vi "test Thermal Chamber Response Simulator_Init-Init.vi"(8 "error in (no error)":errorcluster, 11 "TestCase in":refnum<class "Thermal Chamber Response Simulator_Init.lvclass">) -> (0 "error out":errorcluster, 3 "TestCase out":refnum<class "Thermal Chamber Response Simulator_Init.lvclass">)   [LabVIEW 2018, in "Thermal Chamber Response Simulator_Init.lvclass"]
uses:
  Thermal Chamber Response Simulator_Init.lvclass
  Libraries/Thermal Chamber Response Simulator/Thermal Chamber Response Simulator.lvlib
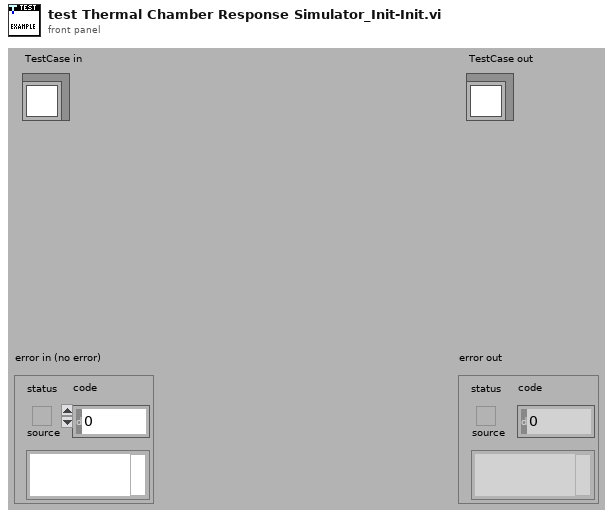
[diagram p1: front panel]
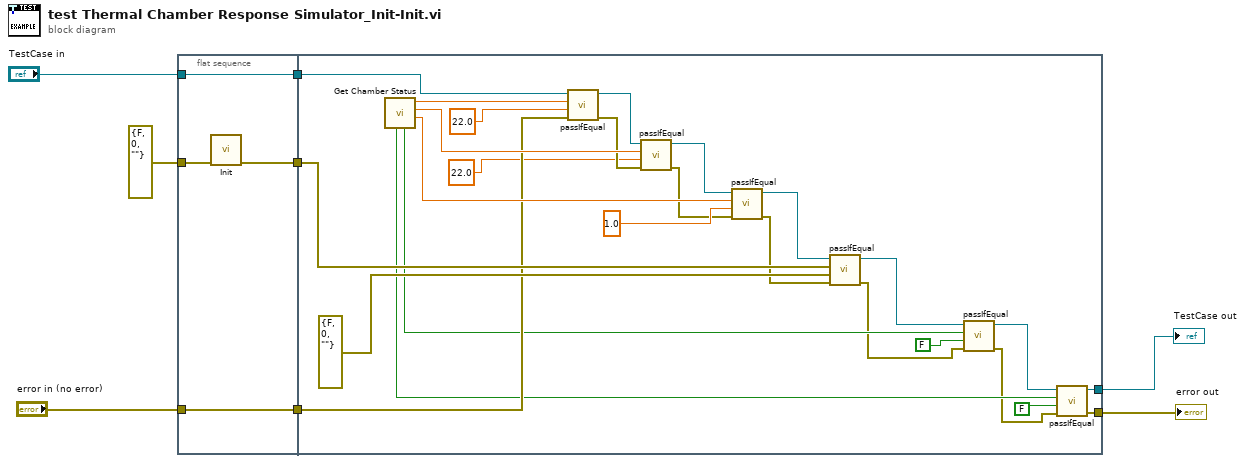
[diagram p0: block diagram]
diagram:
  n1 = flat-sequence {
    tunnel: errorcluster {"status"=FALSE, "code"=0, "source"=""} ("error in (no error)") -> [w12]
    tunnel: [w11] -> w7
    tunnel: "error in (no error)" -> [w10]
    tunnel: [w10] -> w6
    tunnel: [w9] -> w4
    tunnel: "TestCase in" -> [w9]
    tunnel: w7 -> [w38]
    tunnel: w6 -> [w27]
    tunnel: w4 -> [w31]
    tunnel: [w15] -> w2
    tunnel: [w14] -> w1
    frame #0 {
      n2 = call "Init.vi"("error in (no error)"=w12) -> ("error out"=w11:errorcluster)  [unwired: 10 in]
    }
    frame #1 {
      n3 = call "Get Chamber Status.vi"() -> ("Ramp Rate (deg C / second)"=w33:dbl, "Temperature Set Point (deg C)"=w35:dbl, "Actual Temperature"=w36:dbl, "Application Exit"=w23:bool, "Heater State"=w19:bool)  [unwired: 6 in, 1 out]
      n4 = call-dynamic "passIfEqual.vi"("error in (no error)"=w27, "y"=22.0 ("Actual Temperature"), "x"=w36, "TestCase in"=w31) -> ("error out"=w26:errorcluster, "TestCase out"=w30:refnum<class "Thermal Chamber Response Simulator_Init.lvclass">)  [unwired: 6 in]
      n5 = call-dynamic "passIfEqual.vi"("error in (no error)"=w26, "y"=22.0 ("Actual Temperature"), "x"=w35, "TestCase in"=w30) -> ("error out"=w25:errorcluster, "TestCase out"=w29:refnum<class "Thermal Chamber Response Simulator_Init.lvclass">)  [unwired: 6 in]
      n6 = call-dynamic "passIfEqual.vi"("error in (no error)"=w25, "y"=1.0 ("Actual Temperature"), "x"=w33, "TestCase in"=w29) -> ("error out"=w24:errorcluster, "TestCase out"=w28:refnum<class "Thermal Chamber Response Simulator_Init.lvclass">)  [unwired: 6 in]
      n7 = call-dynamic "passIfEqual.vi"("error in (no error)"=w24, "y"=errorcluster {"status"=FALSE, "code"=0, "source"=""} ("error out"), "x"=w38, "TestCase in"=w28) -> ("error out"=w17:errorcluster, "TestCase out"=w22:refnum<class "Thermal Chamber Response Simulator_Init.lvclass">)  [unwired: 6 in]
      n8 = call-dynamic "passIfEqual.vi"("error in (no error)"=w17, "y"=FALSE ("Application Exit"), "x"=w23, "TestCase in"=w22) -> ("error out"=w16:errorcluster, "TestCase out"=w18:refnum<class "Thermal Chamber Response Simulator_Init.lvclass">)  [unwired: 6 in]
      n9 = call-dynamic "passIfEqual.vi"("error in (no error)"=w16, "y"=FALSE ("Application Exit"), "x"=w19, "TestCase in"=w18) -> ("error out"=w15:errorcluster, "TestCase out"=w14:refnum<class "Thermal Chamber Response Simulator_Init.lvclass">)  [unwired: 6 in]
    }
  }
  "error out" <- w2
  "TestCase out" <- w1
